vi "test_Multiple Static Single Channel Command-Response messages using Trigger.vi"(8 "error in (no error)":errorcluster, 11 "TestCase in":refnum<class "Instrument Addon Common System Tests.lvclass">) -> (0 "error out":errorcluster, 3 "TestCase out":refnum<class "Instrument Addon Common System Tests.lvclass">)   [LabVIEW 2019, in "Instrument Addon Common System Tests.lvclass"]
uses:
  Instrument Addon Common System Tests.lvclass
  C:/Program Files (x86)/National Instruments/LabVIEW 2019/vi.lib/NI/VeriStand Custom Device Testing Tools/VeriStandTestCase/VeriStandTestCase.lvclass
  <vilib>/addons/_JKI Toolkits/VI Tester/TestCase.llb/TestCase.lvclass
  C:/Program Files (x86)/National Instruments/LabVIEW 2019/vi.lib/addons/_JKI Toolkits/VI Tester/TestCase.llb/TestCase.lvclass
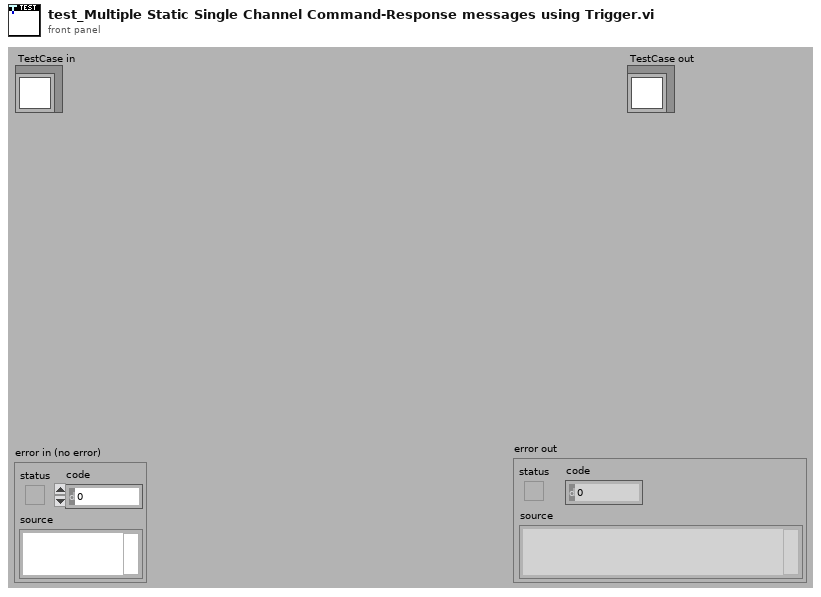
[diagram p1: front panel]
types:
  T1 = typedef "NI_VS Workspace ExecutionAPI.lvlib/WorkspaceAPI.ctl" = refnum<k24>
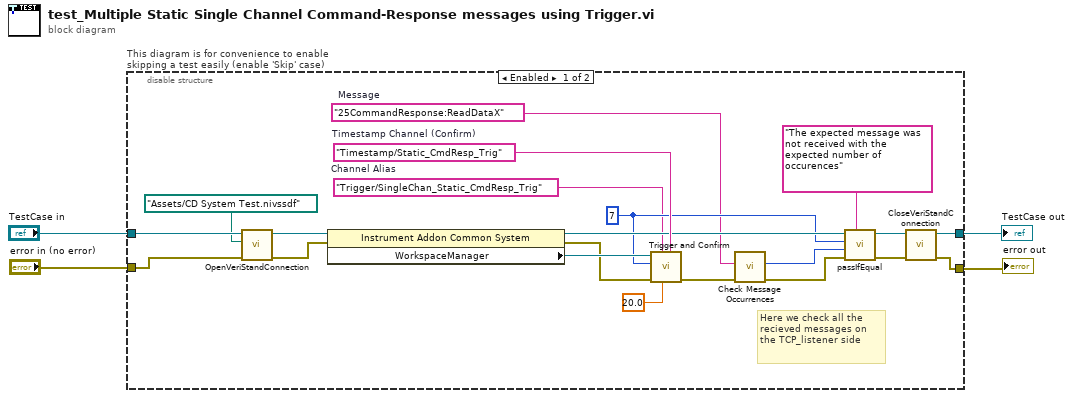
[diagram p0: block diagram]
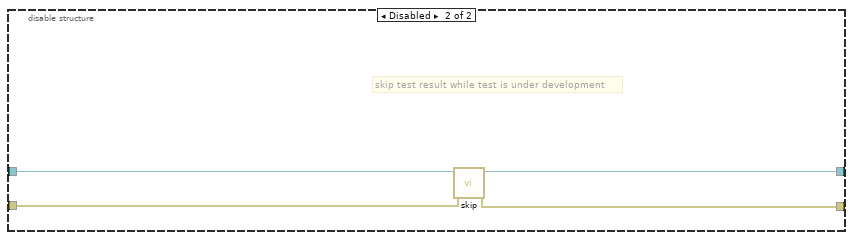
[diagram p2: hidden frame]
diagram:
  n1 = disable-structure "This diagram is for convenience to enable skipping a test easily (enable 'Skip' case)" shown="Enabled" {
    disable-tunnel: "TestCase in" -> [w23 w29]
    disable-tunnel: [w24 w27] -> w2
    disable-tunnel: [w25 w28] -> w1
    disable-tunnel: "error in (no error)" -> [w21 w26]
    frame Enabled {
      w5 = "25CommandResponse:ReadDataX"  # Message
      w6 = "Trigger/SingleChan_Static_CmdResp_Trig"  # Channel Alias
      w9 = 7
      w17 = "Timestamp/Static_CmdResp_Trig"  # Timestamp Channel (Confirm)
      # "Here we check all the recieved messages on the TCP_listener side"
      n2 = call-dynamic "OpenVeriStandConnection.vi"("error in (no error)"=w21, "System Definition File"=path "Assets/CD System Test.nivssdf", "VeriStand Test Case in"=w23) -> ("error out"=w20:errorcluster, "VeriStand Test Case out"=w22:refnum<class "Instrument Addon Common System Tests.lvclass">)  [unwired: 6 in, 1 out]
      n3 = property class="Instrument Addon Common System "(reference=w22, error in=w20) -> (reference out=w12:refnum<class "Instrument Addon Common System Tests.lvclass">, error out=w16:errorcluster, "WorkspaceManager"=w18:T1)
      n4 = call "Trigger and Confirm.vi"("Timestamp Channel (Confirm)"=w17, "Timeout (s)"=20.0, "Trigger Channel"=w6, "error in (no error)"=w16, "Number of Triggers"=w9, "WorkspaceManager in"=w18) -> ("error out"=w15:errorcluster)  [unwired: 4 in, 1 out]
      n5 = call "Check Message Occurrences.vi"("error in (no error)"=w15, "Message"=w5) -> ("error IO"=w13:errorcluster, "Occurences"=w8:i32)  [unwired: 8 in]
      n6 = call-dynamic "passIfEqual.vi"("custom report message (\"\")"="The expected message was not received with the expected number of occurences" ("custom report message (\"\")"), "error in (no error)"=w13, "y"=w8, "x"=w9, "TestCase in"=w12) -> ("error out"=w10:errorcluster, "TestCase out"=w11:refnum<class "Instrument Addon Common System Tests.lvclass">)  [unwired: 5 in]
      n7 = call-dynamic "CloseVeriStandConnection.vi"("error in (no error)"=w10, "VeriStand Test Case in"=w11) -> ("error out"=w25:errorcluster, "VeriStand Test Case out"=w24:refnum<class "Instrument Addon Common System Tests.lvclass">)  [unwired: 8 in]
    }
    frame Disabled {
      # "skip test result while test is under development"
      n8 = call <vilib>:"skip.vi"("error in (no error)"=w26, "TestCase in"=w29) -> ("error out"=w28:errorcluster, "TestCase out"=w27:refnum<class "Instrument Addon Common System Tests.lvclass">)  [unwired: 8 in]
    }
  }
  "error out" <- w1
  "TestCase out" <- w2
